vi "Begin.vi"() -> (0 "error out":errorcluster)   [LabVIEW 2013]
doc: "Called before other user functions, this VI is expected to open initial I/O refnums, load in file data, and do all program initialization. Notice that the <B>error out</B> terminal is simply used for data flow. Wiring it to other structures or subVIs ensures that this VI runs first."
uses:
  <vilib>/Rock Robotics/WPI/SafetyOutput/WPI_SafetyOutputConfigMenu.ctl
  <vilib>/Rock Robotics/WPI/DriverStation/WPI_DriverStationRobotMode2.ctl
  <vilib>/Rock Robotics/WPI/Joystick/WPI_JoystickDeviceEnum.ctl
  <vilib>/Rock Robotics/WPI/Encoder/WPI_EncoderType.ctl
  <vilib>/Rock Robotics/SystemInterfaces/DIO/FPGA_DIOChannel.ctl
  <vilib>/Rock Robotics/SystemInterfaces/AI/FPGA_AIGyroChannel.ctl
  <vilib>/Rock Robotics/WPI/Solenoid/WPI_SolenoidChannel.ctl
  <vilib>/Rock Robotics/SystemInterfaces/DIO/FPGA_DIOPWMChannel.ctl
  Robot Global Data.vi
  <vilib>/Rock Robotics/WPI/Counter/WPI_CounterDigitalInputToDigitalSource.vi
  <vilib>/Rock Robotics/WPI/Solenoid/WPI_SolenoidOpenSingle.vi
  <vilib>/Rock Robotics/WPI/MotorControl/WPI_MotorControlOpen Victor.vi
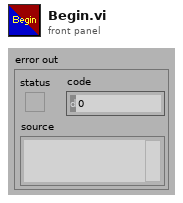
[diagram p1: front panel]
types:
  T1 = typedef "FPGA_DIOPWMChannel.ctl" = enum8{"PWM 1", "PWM 2", "PWM 3", "PWM 4", "PWM 5", "PWM 6", "PWM 7", "PWM 8", "PWM 9", "PWM 10", "Invalid"}
  T2 = typedef "WPI_SolenoidChannel.ctl" = enum8{"Solenoid 1", "Solenoid 2", "Solenoid 3", "Solenoid 4", "Solenoid 5", "Solenoid 6", "Solenoid 7", "Solenoid 8", "Invalid"}
  T3 = typedef "FPGA_DIOChannel.ctl" = enum8{"DIO 1", "DIO 2", "DIO 3", "DIO 4", "DIO 5", "DIO 6", "DIO 7", "DIO 8", "DIO 9", "DIO 10", "DIO 11", "DIO 12", "DIO 13", "DIO 14", "Invalid"}
  T4 = typedef "WPI_EncoderType.ctl" = enum16{"1x", "2x", "4x"}
  T5 = typedef "WPI_JoystickDeviceEnum.ctl" = enum16{"USB 1", "USB 2", "USB 3", "USB 4", "Kinect 1", "Kinect 2"}
  T6 = typedef "FPGA_AIGyroChannel.ctl" = enum8{"AI 1", "AI 2", "Invalid"}
  T7 = typedef "WPI_DriverStationRobotMode2.ctl" = enum16{"Autonomous Disabled", "Autonomous Enabled", "Teleop Disabled", "Teleop Enabled", "Timeout", "Finish", "Test Disabled", "Test Enabled"}
  T8 = typedef "WPI_SafetyOutputConfigMenu.ctl" = enum16{"Enable", "Disable"}
  T9 = typedef "WPI_RobotDriveDevRef.ctl" = cluster{"DevStatus":errorcluster, "Motors[]":T10[], "Square Inputs":bool, "Max Output":dbl, "Isochronous":bool}
  T10 = typedef "WPI_MotorControlDeviceRef.ctl" = cluster{"DeviceStatus":errorcluster, "Type":enum16{"PWM", "CAN"}, "PWM":cluster{"Digital Module":T11, "PWM Channel":T1, "DeadBand":T12}, "CAN":cluster{"Device Number":u8, "Control Mode":T13, "Semaphore":T14, "Max Vout":dbl}, "Invert":bool, "TransformRef":T15, "InvTransformRef":T15}
  T11 = typedef "FPGA_TypedefDigitalModule.ctl" = enum16{"Digital Module 1", "Digital Module 2"}
  T12 = typedef "WPI_PWMDeadband.ctl" = cluster{"Name":string, "maxPositivePwm":i32, "minPositivePwm":i32, "centerPwm":i32, "maxNegativePwm":i32, "minNegativePwm":i32, "angularRange":u16}
  T13 = typedef "WPI_CANJaguar_ControlMode.ctl" = enum8{"Percent VBus", "Current", "Speed", "Position", "Voltage"}
  T14 = typedef "Semaphore RefNum" = refnum<k1>
  T15 = typedef "WPI_PWMTransform_ConPane.ctl" = refnum<vi>
  T16 = typedef "WPI_JoystickDevRef.ctl" = cluster{"Device":T5}
  T17 = typedef "WPI_SolenoidDevRef.ctl" = cluster{"DevStatus":errorcluster, "Solenoid Module":T18, "Forward Solenoid Channel":T2, "Reverse Solenoid Channel":T2}
  T18 = typedef "FPGA_TypedefSolenoidModule.ctl" = enum16{"Solenoid Module 1", "Solenoid Module 2"}
  T19 = typedef "WPI_DigitalInputDevRef.ctl" = cluster{"DevStatus":errorcluster, "DIO Channel":T3, "Digital Module":T11}
  T20 = typedef "WPI_GyroDevRef.ctl" = cluster{"DevStatus":errorcluster, "Analog Module":T21, "Analog Channel":T22, "Offset":dbl, "Gain (VoltsPerDegree/Second)":dbl}
  T21 = typedef "FPGA_TypedefAnalogModule.ctl" = enum16{"Analog Module 1", "Analog Module 2"}
  T22 = typedef "FPGA_AIChannel.ctl" = enum8{"AI 1", "AI 2", "AI 3", "AI 4", "AI 5", "AI 6", "AI 7", "AI 8", "Invalid"}
  T23 = typedef "FPGA_CounterEncoderSourceConvertionLVSourceType.ctl" = cluster{"DevStatus":errorcluster, "AnalogTriggerMode?":bool, "DigitalMode":cluster{"Digital Module":T11, "DIO Channel":T24}, "AnalogTriggerMode":cluster{"AnalogTriggerIndex":T25, "OutputType":T26}}
  T24 = typedef "FPGA_DIODigitalSourceChannel.ctl" = enum8{"DIO 1", "DIO 2", "DIO 3", "DIO 4", "DIO 5", "DIO 6", "DIO 7", "DIO 8", "DIO 9", "DIO 10", "DIO 11", "DIO 12", "DIO 13", "DIO 14", "Disabled"}
  T25 = typedef "FPGA_AnalogTriggerIndex.ctl" = enum8{"Trig 0", "Trig 1", "Trig 2", "Trig 3", "Trig 4", "Trig 5", "Trig 6", "Trig 7", "Invalid"}
  T26 = typedef "FPGA_AnalogTriggerOutType.ctl" = enum16{"InWindow", "TriggerState", "Rising", "Falling"}
  T27 = typedef "WPI_EncoderDevRef.ctl" = cluster{"DevStatus":errorcluster, "EncoderIndex":T28, "CounterIndex":T29, "DistancePerCount":dbl, "Decoding Type":T4}
  T28 = typedef "FPGA_EncoderIdx.ctl" = enum8{"Enc 0", "Enc 1", "Enc 2", "Enc 3", "Invalid"}
  T29 = typedef "FPGA_CounterCtrSystemIndex.ctl" = enum8{"Ctr 0", "Ctr 1", "Ctr 2", "Ctr 3", "Ctr 4", "Ctr 5", "Ctr 6", "Ctr 7", "Invalid"}
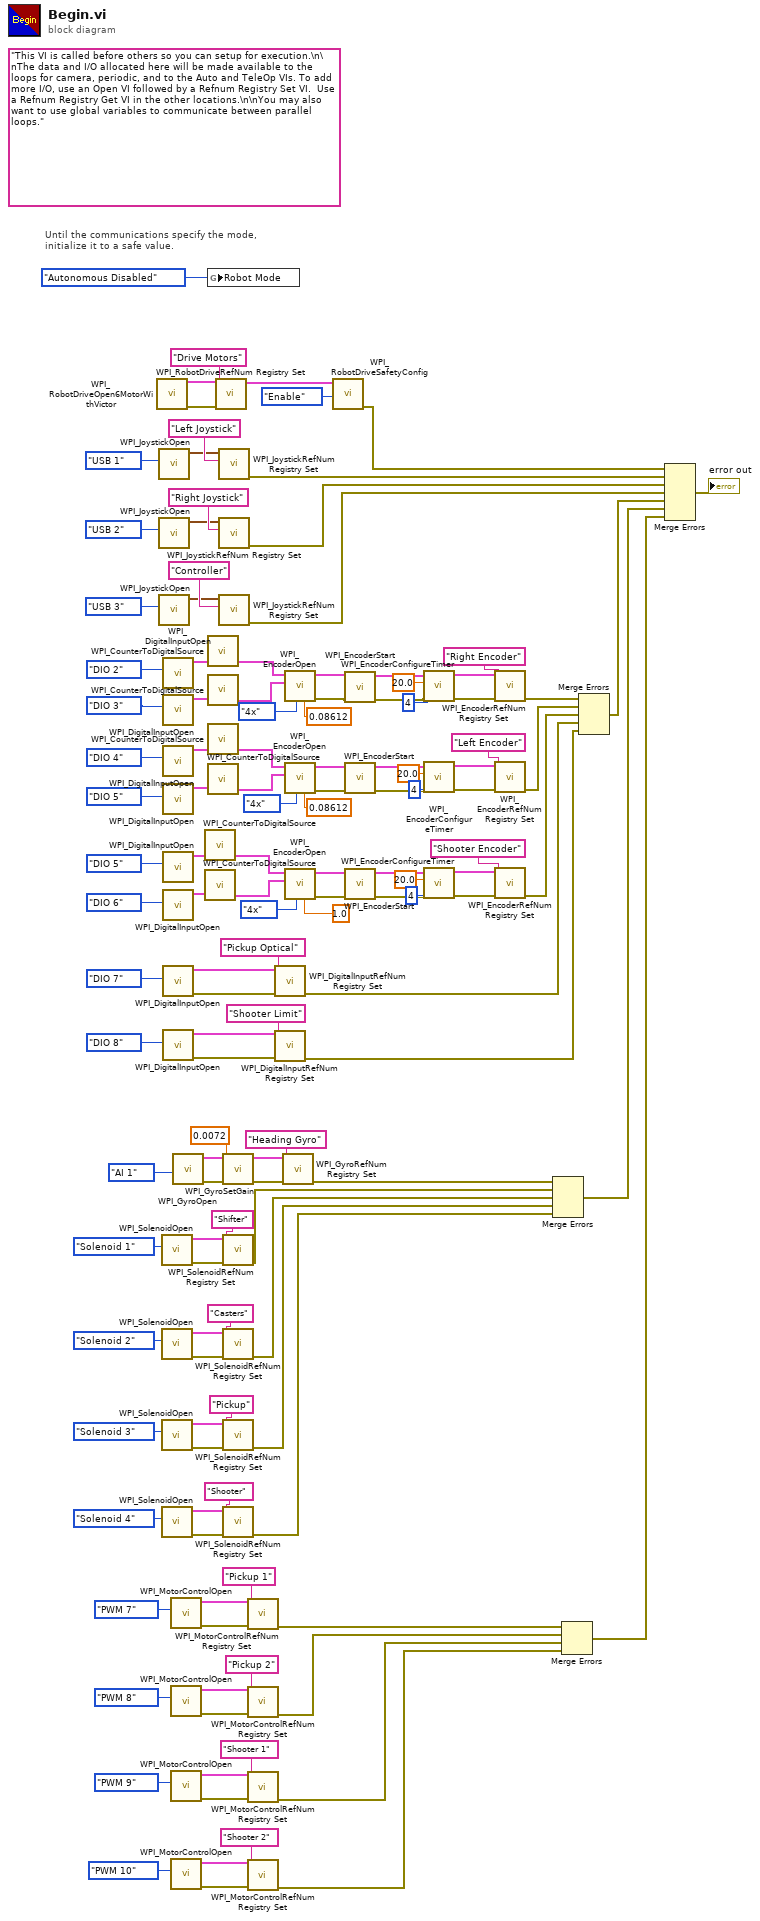
[diagram p0: block diagram]
diagram:
  (unwired) "This VI is called before others so you can setup for execution.\n\nThe data and I/O allocated here will be made available to the loops for camera, periodic, and to the Auto and TeleOp VIs. To add more I/O, use an Open VI followed by a Refnum Registry Set VI.  Use a Refnum Registry Get VI in the other locations.\n\nYou may also want to use global variables to communicate between parallel loops."
  # "Until the communications specify the mode,\ninitialize it to a safe value."
  n1 = call "WPI_RobotDriveOpen6MotorWithVictor.vi"() -> ("RobotDriveDevRef"=w120:T9, "error out"=w121:errorcluster)  [unwired: 14 in]
  n2 = call <vilib>:"WPI_JoystickOpen.vi"("JoystickDevice"=WPI_JoystickDeviceEnum."USB 1") -> ("JoystickDevRef"=w130:T16)  [unwired: 10 in]
  n3 = call <vilib>:"WPI_JoystickOpen.vi"("JoystickDevice"=WPI_JoystickDeviceEnum."USB 2") -> ("JoystickDevRef"=w127:T16)  [unwired: 10 in]
  n4 = call <vilib>:"WPI_JoystickOpen.vi"("JoystickDevice"=WPI_JoystickDeviceEnum."USB 3") -> ("JoystickDevRef"=w87:T16)  [unwired: 10 out]
  n5 = call-poly <vilib>:"WPI_SolenoidOpen.vi"("Solenoid Channel"=WPI_SolenoidChannel."Solenoid 1") -> ("error out"=w84:errorcluster, "SolenoidDevRef"=w71:T17)  [unwired: 9 in]
  n6 = call-poly <vilib>:"WPI_SolenoidOpen.vi"("Solenoid Channel"=WPI_SolenoidChannel."Solenoid 2") -> ("error out"=w60:errorcluster, "SolenoidDevRef"=w59:T17)  [unwired: 9 in]
  n7 = call-poly <vilib>:"WPI_SolenoidOpen.vi"("Solenoid Channel"=WPI_SolenoidChannel."Solenoid 3") -> ("error out"=w47:errorcluster, "SolenoidDevRef"=w46:T17)  [unwired: 9 in]
  n8 = call-poly <vilib>:"WPI_SolenoidOpen.vi"("Solenoid Channel"=WPI_SolenoidChannel."Solenoid 4") -> ("error out"=w16:errorcluster, "SolenoidDevRef"=w15:T17)  [unwired: 9 in]
  n9 = call <vilib>:"WPI_DigitalInputOpen.vi"("DIO Channel"=FPGA_DIOChannel."DIO 2") -> ("DigitalInputDevRef"=w105:T19)  [unwired: 2 in, 8 out]
  n10 = call <vilib>:"WPI_DigitalInputOpen.vi"("DIO Channel"=FPGA_DIOChannel."DIO 3") -> ("DigitalInputDevRef"=w101:T19)  [unwired: 2 in, 8 out]
  n11 = call <vilib>:"WPI_DigitalInputOpen.vi"("DIO Channel"=FPGA_DIOChannel."DIO 4") -> ("DigitalInputDevRef"=w98:T19)  [unwired: 2 in, 8 out]
  n12 = call <vilib>:"WPI_DigitalInputOpen.vi"("DIO Channel"=FPGA_DIOChannel."DIO 5") -> ("DigitalInputDevRef"=w96:T19)  [unwired: 2 in, 8 out]
  n13 = call <vilib>:"WPI_DigitalInputOpen.vi"("DIO Channel"=FPGA_DIOChannel."DIO 5") -> ("DigitalInputDevRef"=w36:T19)  [unwired: 2 in, 8 out]
  n14 = call <vilib>:"WPI_DigitalInputOpen.vi"("DIO Channel"=FPGA_DIOChannel."DIO 6") -> ("DigitalInputDevRef"=w34:T19)  [unwired: 2 in, 8 out]
  n15 = call <vilib>:"WPI_DigitalInputOpen.vi"("DIO Channel"=FPGA_DIOChannel."DIO 7") -> ("error out"=w23:errorcluster, "DigitalInputDevRef"=w22:T19)  [unwired: 2 in, 7 out]
  n16 = call <vilib>:"WPI_DigitalInputOpen.vi"("DIO Channel"=FPGA_DIOChannel."DIO 8") -> ("error out"=w20:errorcluster, "DigitalInputDevRef"=w21:T19)  [unwired: 2 in, 7 out]
  n17 = call-poly <vilib>:"WPI_MotorControlOpen.vi"("PWM Channel"=FPGA_DIOPWMChannel."PWM 7") -> ("error out"=w67:errorcluster, "MotorControlDeviceRef"=w68:T10)  [unwired: 9 in]
  n18 = call-poly <vilib>:"WPI_MotorControlOpen.vi"("PWM Channel"=FPGA_DIOPWMChannel."PWM 8") -> ("error out"=w63:errorcluster, "MotorControlDeviceRef"=w64:T10)  [unwired: 9 in]
  n19 = call-poly <vilib>:"WPI_MotorControlOpen.vi"("PWM Channel"=FPGA_DIOPWMChannel."PWM 9") -> ("error out"=w8:errorcluster, "MotorControlDeviceRef"=w9:T10)  [unwired: 9 in]
  n20 = call-poly <vilib>:"WPI_MotorControlOpen.vi"("PWM Channel"=FPGA_DIOPWMChannel."PWM 10") -> ("error out"=w4:errorcluster, "MotorControlDeviceRef"=w5:T10)  [unwired: 9 in]
  n21 = call <vilib>:"WPI_GyroOpen.vi"("Analog Channel"=FPGA_AIGyroChannel."AI 1") -> ("error out"=w53:errorcluster, "GyroDevRef"=w52:T20)  [unwired: 5 in, 4 out]
  n22 = call-poly <vilib>:"WPI_CounterToDigitalSource.vi"("DigitalInputDevRef"=w36) -> ("Digital Source"=w33:T23)  [unwired: 6 out]
  n23 = call-poly <vilib>:"WPI_CounterToDigitalSource.vi"("DigitalInputDevRef"=w34) -> ("Digital Source"=w32:T23)  [unwired: 6 out]
  n24 = global write "Robot Global Data.vi" "Robot Mode"(WPI_DriverStationRobotMode2."Autonomous Disabled" ("Robot Mode")) -> ()
  n25 = call-poly <vilib>:"WPI_CounterToDigitalSource.vi"("DigitalInputDevRef"=w105) -> ("Digital Source"=w106:T23)  [unwired: 6 out]
  n26 = call-poly <vilib>:"WPI_CounterToDigitalSource.vi"("DigitalInputDevRef"=w101) -> ("Digital Source"=w102:T23)  [unwired: 6 out]
  n27 = call-poly <vilib>:"WPI_CounterToDigitalSource.vi"("DigitalInputDevRef"=w98) -> ("Digital Source"=w95:T23)  [unwired: 6 out]
  n28 = call-poly <vilib>:"WPI_CounterToDigitalSource.vi"("DigitalInputDevRef"=w96) -> ("Digital Source"=w94:T23)  [unwired: 6 out]
  n29 = call <vilib>:"WPI_RobotDriveRefNum Registry Set.vi"("error in (no error)"=w121, "refnum name"="Drive Motors", "RobotDriveDevRef"=w120) -> ("RobotDriveDevRef"=w134:T9)  [unwired: 8 out]
  n30 = call <vilib>:"WPI_JoystickRefNum Registry Set.vi"("refnum name"="Left Joystick", "JoystickDevRef"=w130) -> ("error out"=w124:errorcluster)  [unwired: 8 in, 1 out]
  n31 = call <vilib>:"WPI_JoystickRefNum Registry Set.vi"("refnum name"="Right Joystick", "JoystickDevRef"=w127) -> ("error out"=w123:errorcluster)  [unwired: 8 in, 1 out]
  n32 = call <vilib>:"WPI_JoystickRefNum Registry Set.vi"("refnum name"="Controller", "JoystickDevRef"=w87) -> ("error out"=w86:errorcluster)  [unwired: 1 in, 8 out]
  n33 = call <vilib>:"WPI_GyroSetGain.vi"("error in (no error)"=w53, "Gain (VoltsPerDegree/Second)"=0.0072, "GyroDevRef"=w52) -> ("error out"=w49:errorcluster, "GyroDevRef"=w50:T20)  [unwired: 7 in]
  n34 = call <vilib>:"WPI_SolenoidRefNum Registry Set.vi"("error in (no error)"=w84, "refnum name"="Shifter", "SolenoidDevRef"=w71) -> ("error out"=w74:errorcluster)  [unwired: 7 in, 1 out]
  n35 = call <vilib>:"WPI_SolenoidRefNum Registry Set.vi"("error in (no error)"=w60, "refnum name"="Casters", "SolenoidDevRef"=w59) -> ("error out"=w57:errorcluster)  [unwired: 7 in, 1 out]
  n36 = call <vilib>:"WPI_SolenoidRefNum Registry Set.vi"("error in (no error)"=w47, "refnum name"="Pickup", "SolenoidDevRef"=w46) -> ("error out"=w44:errorcluster)  [unwired: 7 in, 1 out]
  n37 = call <vilib>:"WPI_SolenoidRefNum Registry Set.vi"("error in (no error)"=w16, "refnum name"="Shooter", "SolenoidDevRef"=w15) -> ("error out"=w13:errorcluster)  [unwired: 7 in, 1 out]
  n38 = call <vilib>:"WPI_MotorControlRefNum Registry Set.vi"("error in (no error)"=w67, "refnum name"="Pickup 1", "MotorControlDevRef"=w68) -> ("error out"=w55:errorcluster)  [unwired: 7 in, 1 out]
  n39 = call <vilib>:"WPI_MotorControlRefNum Registry Set.vi"("error in (no error)"=w63, "refnum name"="Pickup 2", "MotorControlDevRef"=w64) -> ("error out"=w56:errorcluster)  [unwired: 7 in, 1 out]
  n40 = call <vilib>:"WPI_MotorControlRefNum Registry Set.vi"("error in (no error)"=w8, "refnum name"="Shooter 1", "MotorControlDevRef"=w9) -> ("error out"=w2:errorcluster)  [unwired: 7 in, 1 out]
  n41 = call <vilib>:"WPI_MotorControlRefNum Registry Set.vi"("error in (no error)"=w4, "refnum name"="Shooter 2", "MotorControlDevRef"=w5) -> ("error out"=w1:errorcluster)  [unwired: 7 in, 1 out]
  n42 = call <vilib>:"WPI_DigitalInputRefNum Registry Set.vi"("error in (no error)"=w23, "refnum name"="Pickup Optical", "DigitalInputDevRef"=w22) -> ("error out"=w12:errorcluster)  [unwired: 7 in, 1 out]
  n43 = call <vilib>:"WPI_DigitalInputRefNum Registry Set.vi"("error in (no error)"=w20, "refnum name"="Shooter Limit", "DigitalInputDevRef"=w21) -> ("error out"=w11:errorcluster)  [unwired: 7 in, 1 out]
  n44 = call <vilib>:"WPI_GyroRefNum Registry Set.vi"("error in (no error)"=w49, "refnum name"="Heading Gyro", "GyroDevRef"=w50) -> ("error out"=w75:errorcluster)  [unwired: 8 out]
  n45 = call <vilib>:"WPI_EncoderOpen.vi"("DistancePerCount"=0.08612, "Decoding Type"=WPI_EncoderType."4x", "BSource"=w102, "ASource"=w106) -> ("error out"=w83:errorcluster, "EncoderDevRef"=w119:T27)  [unwired: 4 in, 2 out]
  n46 = call <vilib>:"WPI_EncoderOpen.vi"("DistancePerCount"=0.08612, "Decoding Type"=WPI_EncoderType."4x", "BSource"=w94, "ASource"=w95) -> ("error out"=w80:errorcluster, "EncoderDevRef"=w116:T27)  [unwired: 4 in, 2 out]
  n47 = call <vilib>:"WPI_EncoderOpen.vi"("DistancePerCount"=1.0, "Decoding Type"=WPI_EncoderType."4x", "BSource"=w32, "ASource"=w33) -> ("error out"=w29:errorcluster, "EncoderDevRef"=w43:T27)  [unwired: 4 in, 2 out]
  n48 = call <vilib>:"WPI_RobotDriveSafetyConfig.vi"("mode"=WPI_SafetyOutputConfigMenu."Enable", "RobotDriveDevRef"=w134) -> ("error out"=w122:errorcluster)  [unwired: 8 in, 1 out]
  n49 = call <vilib>:"WPI_EncoderStart.vi"("error in (no error)"=w83, "EncoderDevRef"=w119) -> ("error out"=w82:errorcluster, "EncoderDevRef"=w118:T27)  [unwired: 8 out]
  n50 = call <vilib>:"WPI_EncoderStart.vi"("error in (no error)"=w80, "EncoderDevRef"=w116) -> ("error out"=w79:errorcluster, "EncoderDevRef"=w115:T27)  [unwired: 8 out]
  n51 = call <vilib>:"WPI_EncoderStart.vi"("error in (no error)"=w29, "EncoderDevRef"=w43) -> ("error out"=w28:errorcluster, "EncoderDevRef"=w42:T27)  [unwired: 8 out]
  n52 = call <vilib>:"WPI_EncoderConfigureTimer.vi"("error in (no error)"=w82, "Number Samples to Average"=u8 4, "Minimum Rate"=20.0, "EncoderDevRef"=w118) -> ("error out"=w81:errorcluster, "EncoderDevRef"=w117:T27)  [unwired: 6 out]
  n53 = call <vilib>:"WPI_EncoderConfigureTimer.vi"("error in (no error)"=w79, "Number Samples to Average"=u8 4, "Minimum Rate"=20.0, "EncoderDevRef"=w115) -> ("error out"=w78:errorcluster, "EncoderDevRef"=w114:T27)  [unwired: 6 out]
  n54 = call <vilib>:"WPI_EncoderConfigureTimer.vi"("error in (no error)"=w28, "Number Samples to Average"=u8 4, "Minimum Rate"=20.0, "EncoderDevRef"=w42) -> ("error out"=w27:errorcluster, "EncoderDevRef"=w41:T27)  [unwired: 6 out]
  n55 = call <vilib>:"WPI_EncoderRefNum Registry Set.vi"("error in (no error)"=w81, "refnum name"="Right Encoder", "EncoderDevRef"=w117) -> ("error out"=w77:errorcluster)  [unwired: 8 out]
  n56 = call <vilib>:"WPI_EncoderRefNum Registry Set.vi"("error in (no error)"=w78, "refnum name"="Left Encoder", "EncoderDevRef"=w114) -> ("error out"=w76:errorcluster)  [unwired: 8 out]
  n57 = call <vilib>:"WPI_EncoderRefNum Registry Set.vi"("error in (no error)"=w27, "refnum name"="Shooter Encoder", "EncoderDevRef"=w41) -> ("error out"=w26:errorcluster)  [unwired: 8 out]
  n58 = Merge Errors(w75, w74, w57, w44, w13) -> (w72:errorcluster)
  n59 = Merge Errors(w55, w56, w2, w1) -> (w54:errorcluster)
  n60 = Merge Errors(w77, w76, w26, w12, w11) -> (w73:errorcluster)
  n61 = Merge Errors(w122, w124, w123, w86, w73, w72, w54) -> (→"error out":errorcluster)
